vi "CAN Jaguar Set Output.vi"(8 "error in (no error)":errorcluster, 10 "Output Set Point":dbl, 11 "CAN Jaguar Ref":T1={"Device Number"=0, "Control Mode"=enum."Percent VBus", "Inverted"=FALSE, "Semaphore"=refnum, "Max Vout"=12.0, "DevStatus"={"status"=FALSE, "code"=0, "source"=""}}) -> (0 "error out":errorcluster, 3 "CAN Jaguar Ref Out":T1={"Device Number"=0, "Control Mode"=enum."Percent VBus", "Inverted"=FALSE, "Semaphore"=refnum, "Max Vout"=12.0, "DevStatus"={"status"=FALSE, "code"=0, "source"=""}})   [LabVIEW 2009, in "CAN.lvlib"]
uses:
  CAN.lvlib
  SubVIs/CAN Jaguar Ref.ctl
  SubVIs/CAN Jaguar Control Mode.ctl
  SubVIs/CAN Token Message IDs.ctl
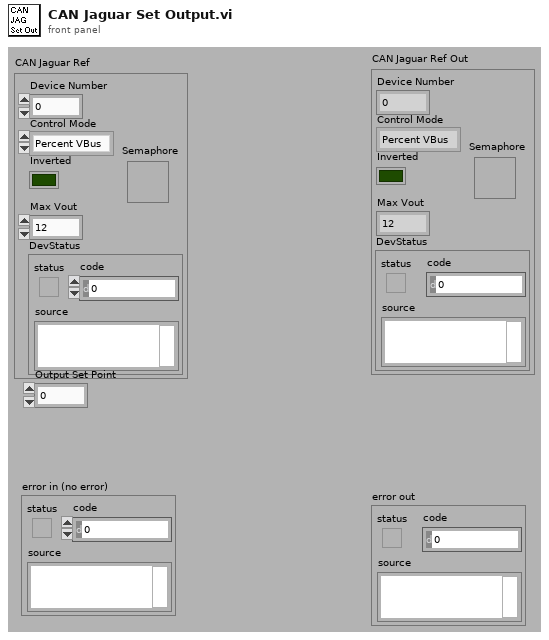
[diagram p1: front panel]
types:
  T1 = typedef "CAN.lvlib/CAN Jaguar Ref.ctl" = cluster{"Device Number":u8, "Control Mode":T2, "Inverted":bool, "Semaphore":T3, "Max Vout":dbl, "DevStatus":errorcluster}
  T2 = typedef "CAN.lvlib/CAN Jaguar Control Mode.ctl" = enum16{"Percent VBus", "Speed", "Position", "Current"}
  T3 = typedef "Semaphore RefNum" = refnum<k1>
  T4 = enum16{"big-endian, network order", "native, host order", "little-endian"}
  T5 = typedef "CAN.lvlib/CAN Token Message IDs.ctl" = u32
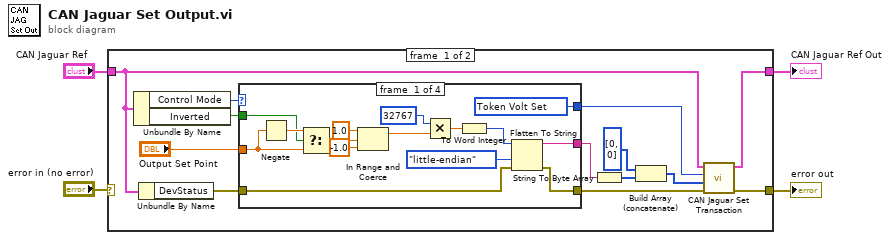
[diagram p0: block diagram]
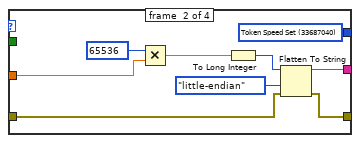
[diagram p2: hidden frame]
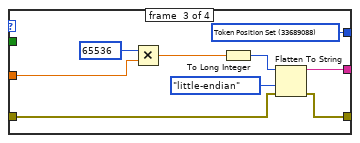
[diagram p3: hidden frame]
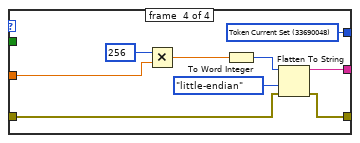
[diagram p4: hidden frame]
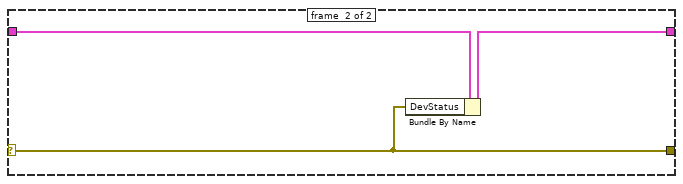
[diagram p5: hidden frame]
diagram:
  n1 = case shown="No Error" "error in (no error)" {
    selector: "error in (no error)" -> [_ w60]
    tunnel: [w7 w60] -> w4
    tunnel: [w8 w61] -> w2
    tunnel: "CAN Jaguar Ref" -> [w5 w62]
    frame #0 {
      n2 = Unbundle By Name(w5) -> ("Control Mode"=w15:T2, "Inverted"=w12:bool)
      n3 = Unbundle By Name(w5) -> ("DevStatus"=w6:errorcluster)
      n4 = case shown="\"Position\"" w15 {
        tunnel: [w32 w41 w50 w59] -> w9
        tunnel: "Output Set Point" -> [w20 w34 w43 w53]
        tunnel: w6 -> [w28 w38 w46 w57]
        tunnel: [w27 w37 w45 w56] -> w11
        tunnel: [w22 w36 w47 w55] -> w13
        tunnel: w12 -> [w19 _ _ _]
        frame #0 {
          w32 = T5 33685824 items=["Token Volt Enable"=33685760, "Token Volt Set"=33685824, "Token Speed Enable"=33686976, "Token Speed Set"=33687040, "Token Position Enable"=33689024, "Token Position Set"=33689088, "Token Current Enable"=33689984, "Token Current Set"=33690048] ("CAN Token Message IDs")
          n5 = Negate(x=w20) -> (-x=w21:dbl)
          n6 = Select(t=w21, s=w19, f=w20) -> (s? t:f=w18:dbl)
          n7 = In Range and Coerce(upper limit=1.0, x=w18, lower limit=-1.0) -> (coerced(x)=w26:dbl)  [unwired: 1 out]
          n8 = Multiply(x=i16 32767, y=w26) -> (x*y=w24:dbl)
          n9 = To Word Integer(number=w24) -> (16bit integer=w23:i16)
          n10 = Flatten To String(anything=w23, byte order (0:big-endian, network order)=T4."little-endian", error in (no error)=w28) -> (data string=w22:string, error out=w27:errorcluster)  [unwired: 2 out]
        }
        frame #1 {
          w41 = T5 33687040 items=["Token Volt Enable"=33685760, "Token Volt Set"=33685824, "Token Speed Enable"=33686976, "Token Speed Set"=33687040, "Token Position Enable"=33689024, "Token Position Set"=33689088, "Token Current Enable"=33689984, "Token Current Set"=33690048] ("CAN Token Message IDs")
          n11 = Multiply(x=u32 65536, y=w34) -> (x*y=w33:dbl)
          n12 = To Long Integer(number=w33) -> (32bit integer=w40:i32)
          n13 = Flatten To String(anything=w40, byte order (0:big-endian, network order)=T4."little-endian", error in (no error)=w38) -> (data string=w36:string, error out=w37:errorcluster)  [unwired: 2 out]
        }
        frame #2 {
          w50 = T5 33689088 items=["Token Volt Enable"=33685760, "Token Volt Set"=33685824, "Token Speed Enable"=33686976, "Token Speed Set"=33687040, "Token Position Enable"=33689024, "Token Position Set"=33689088, "Token Current Enable"=33689984, "Token Current Set"=33690048] ("CAN Token Message IDs")
          n14 = Multiply(x=u32 65536, y=w43) -> (x*y=w42:dbl)
          n15 = To Long Integer(number=w42) -> (32bit integer=w48:i32)
          n16 = Flatten To String(anything=w48, byte order (0:big-endian, network order)=T4."little-endian", error in (no error)=w46) -> (data string=w47:string, error out=w45:errorcluster)  [unwired: 2 out]
        }
        frame #3 {
          w59 = T5 33690048 items=["Token Volt Enable"=33685760, "Token Volt Set"=33685824, "Token Speed Enable"=33686976, "Token Speed Set"=33687040, "Token Position Enable"=33689024, "Token Position Set"=33689088, "Token Current Enable"=33689984, "Token Current Set"=33690048] ("CAN Token Message IDs")
          n17 = Multiply(x=u32 256, y=w53) -> (x*y=w52:dbl)
          n18 = To Word Integer(number=w52) -> (16bit integer=w54:i16)
          n19 = Flatten To String(anything=w54, byte order (0:big-endian, network order)=T4."little-endian", error in (no error)=w57) -> (data string=w55:string, error out=w56:errorcluster)  [unwired: 2 out]
        }
      }
      n20 = String To Byte Array(string=w13) -> (unsigned byte array=w17:u8[])
      n21 = Build Array (concatenate)(u8[] [0, 0] ("data"), w17) -> (w10:u8[])
      n22 = call "CAN Jaguar Set Transaction.vi"("error in"=w11, "Data"=w10, "Message ID"=w9, "CAN Jaguar Ref"=w5) -> ("error out"=w7:errorcluster, "CAN Jaguar Ref Out"=w8:T1)  [unwired: 6 out]
    }
    frame #1 {
      n23 = Bundle By Name(cluster=w62, "DevStatus"=w60) -> (w61:T1)
    }
  }
  "CAN Jaguar Ref Out" <- w2
  "error out" <- w4
